vi "Customized Ini Tokens Folder.vi"() -> (14 "appended path":path)   [LabVIEW 2012]
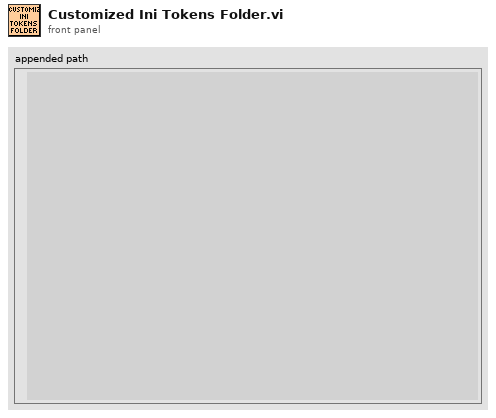
[diagram p1: front panel]
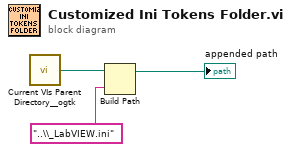
[diagram p0: block diagram]
diagram:
  n1 = call <userlib>:"Current VIs Parent Directory__ogtk.vi"() -> ("Parent Directory (+ Relative)"=w2:path)  [unwired: 5 in]
  n2 = Build Path(base path=w2, name or relative path="..\\_LabVIEW.ini") -> (appended path=→"appended path":path)
